vi "PV ActiveLine - Temperature.vi"(8 "Fehler (Eingang)":errorcluster, 11 "Referenz in":refnum<visa-resource-name>) -> (0 "Cluster (Ausgang)":errorcluster caption="Fehler (Ausgang)", 1 "Temperature":i16, 3 "Referenz out":refnum<visa-resource-name>)   [LabVIEW 2013, in "PV ActiveLine.lvlib"]
doc: "TMP - Temperature Internal temperature of the TPG 36x.\n\nReceive: aa\n\nTemperature (±2 °C) [°C]"
uses:
  <instrlib>/PV ActiveLine/PV ActiveLine.lvlib
panel:
  # "°C"
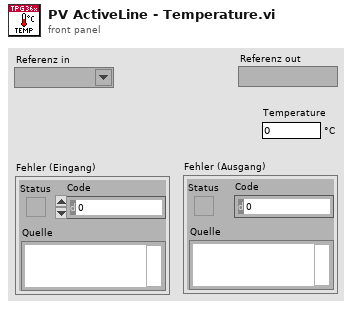
[diagram p1: front panel]
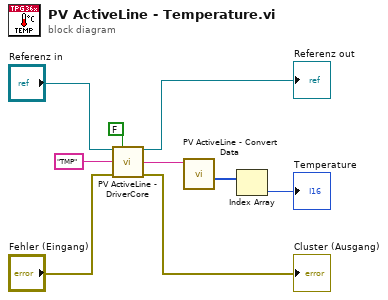
[diagram p0: block diagram]
diagram:
  n1 = call <instrlib>:"PV ActiveLine - DriverCore.vi"("Referenz in"="Referenz in", "Write/Read"=FALSE, "Command"="TMP", "Fehler (Eingang)"="Fehler (Eingang)") -> ("Referenz out"=→"Referenz out":refnum<visa-resource-name>, "String Out"=w3:string, "Cluster (Ausgang)"=→"Cluster (Ausgang)":errorcluster)  [unwired: 9 in]
  n2 = call <instrlib>:"PV ActiveLine - Convert Data.vi"("String in"=w3) -> ("Integer Out"=w2:i32[])  [unwired: 7 in, 3 out]
  n3 = Index Array(array=w2) -> (element=→"Temperature":i32)  [unwired: 1 in]
